vi "Fatal.vi"(8 "Error In":errorcluster, 11 "Message":string) -> (0 "Error Out":errorcluster)   [LabVIEW 2014, in "LV-Logger.lvlib"]
uses:
  LV-Logger.lvlib
  Action.ctl
  Level.ctl
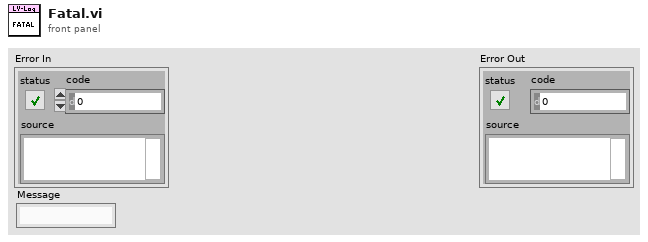
[diagram p1: front panel]
types:
  T1 = typedef "LV-Logger.lvlib/Level.ctl" = enum16{"Fatal", "Error", "Warn", "Info", "Debug", "Trace"}
  T2 = typedef "LV-Logger.lvlib/Action.ctl" = enum16{"Initialize", "Get", "Log", "Shutdown"}
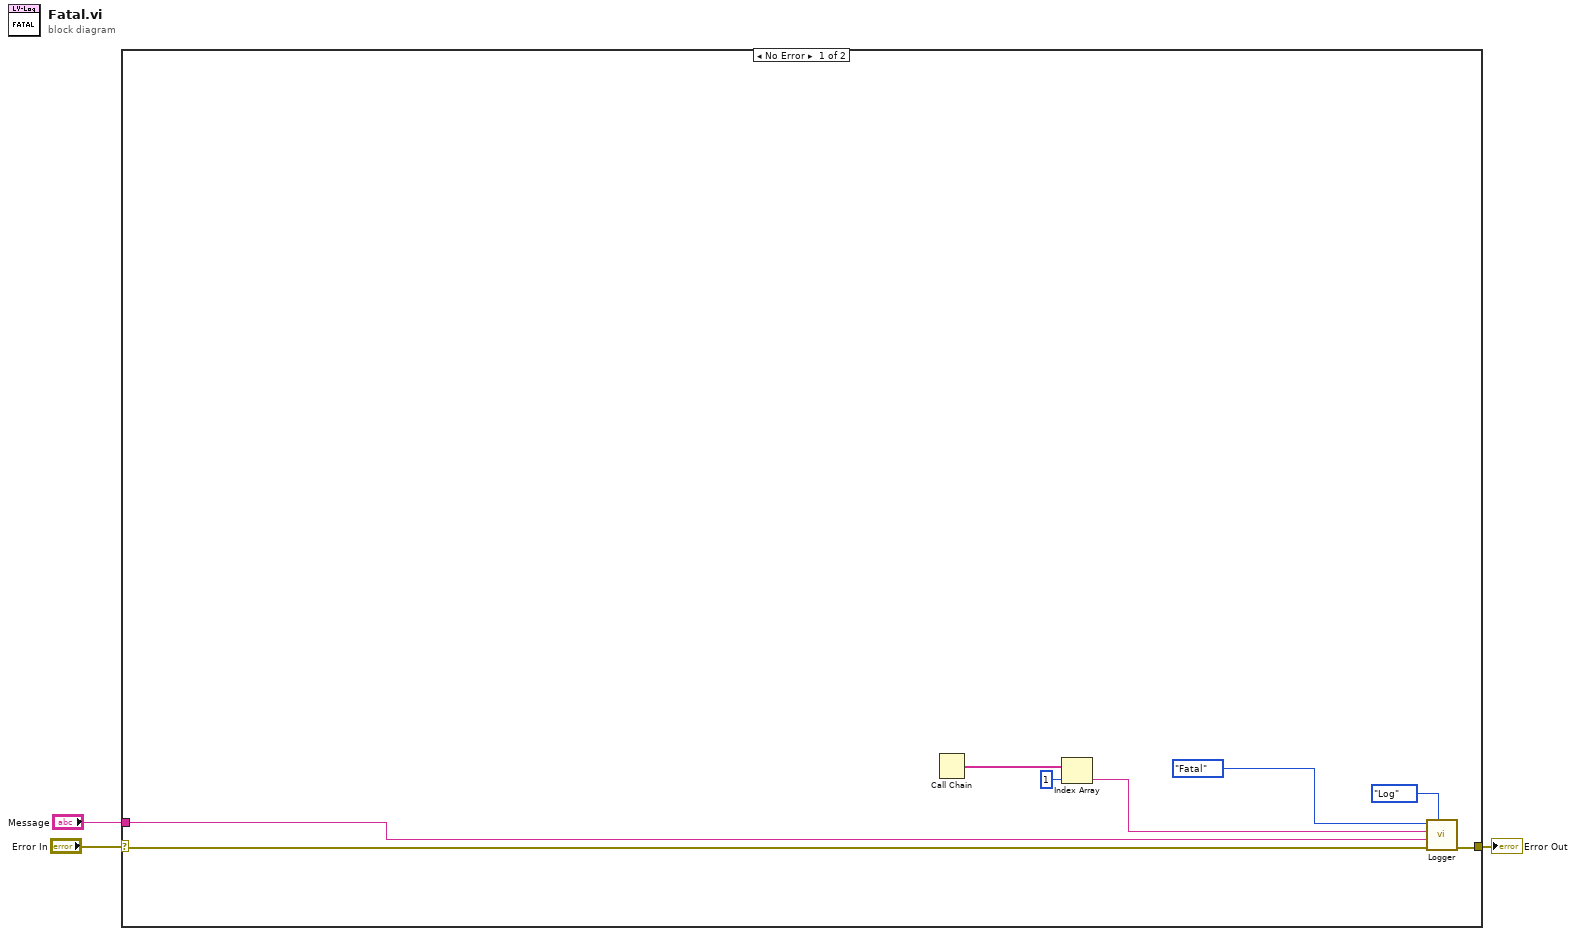
[diagram p0: block diagram]
diagram:
  n1 = case shown="No Error" "Error In" {
    selector: "Error In" -> [w6 w12]
    tunnel: [w5 w12] -> w2
    tunnel: "Message" -> [w4 _]
    frame No Error {
      n2 = Call Chain() -> (call chain=w9:string[])
      n3 = Index Array(array=w9, index=1) -> (element=w7:string)
      n4 = call "Logger.vi"("Action"=Action."Log", "Error In"=w6, "Message"=w4, "Source"=w7, "Level"=Level."Fatal") -> ("Error Out"=w5:errorcluster)  [unwired: 5 in, 1 out]
    }
    frame Error {
    }
  }
  "Error Out" <- w2
